vi "CliCommandReceived.vi"(8 "error in (no error)":errorcluster, 10 "CommandReceived":refnum<class "CommandReceived.lvclass">, 11 "Controller in":refnum<class "Controller.lvclass">) -> (0 "error out":errorcluster, 3 "Controller out":refnum<class "Controller.lvclass">)   [LabVIEW 2022 SP3, in "Controller.lvlib" / "Controller.lvclass"]
uses:
  Controller.lvclass
  Cli/CommandReceived/CommandReceived.lvclass
  Cli/CommandReceived/CommandReceived.lvclass/CommandReceived.ctl
  ArgumentParser/Source/ParsedData/ParsedData.lvclass/ParsedData.ctl
  Cli/CommandReceived/Read ParsedData.vi
  ArgumentParser/Source/ParsedData/Read Arguments.vi
  ArgumentParser/Source/ParsedData/ParsedData.lvclass
  Controller.lvclass/Controller.ctl
  ArgumentParser/Source/ParsedData/_Arguments.ctl
  Cli/Cli Messages/WriteToStdOut Msg/WriteToStdOut Msg.lvclass
  Tcp/DataReceived/DataReceived.lvclass
panel:
  out "Arguments":T1
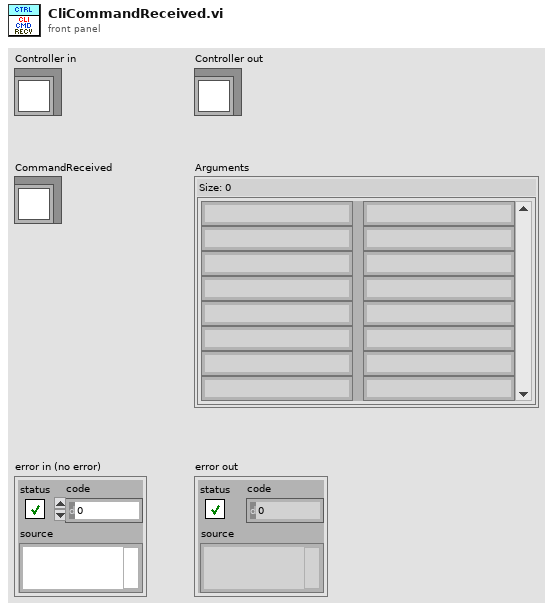
[diagram p1: front panel]
types:
  T1 = typedef "ArgumentParser.lvlib/ParsedData.lvclass/_Arguments.ctl" = map{string, string}
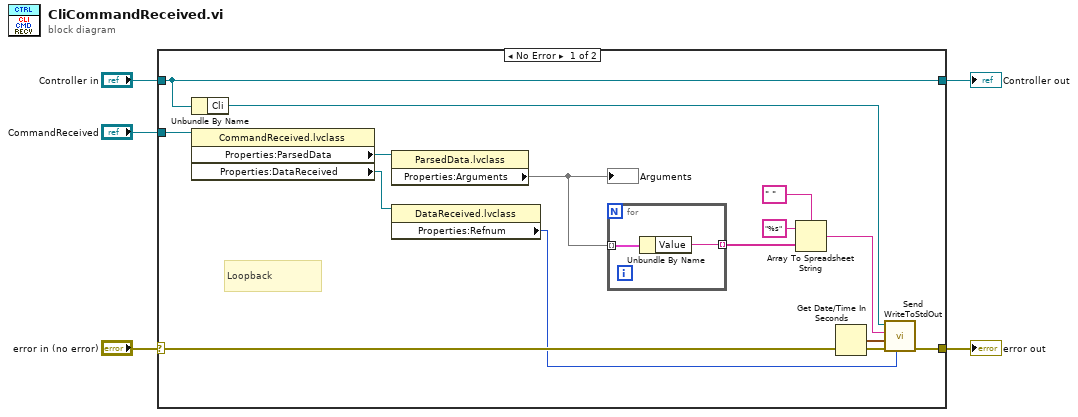
[diagram p0: block diagram]
diagram:
  n1 = case shown="No Error" "error in (no error)" {
    selector: "error in (no error)" -> [w16 w23]
    tunnel: "CommandReceived" -> [w19 _]
    tunnel: [w15 w23] -> w3
    tunnel: "Controller in" -> [w17 w22]
    tunnel: [w17 w22] -> w1
    frame No Error {
      # "Loopback"
      n2 = Unbundle By Name(w17) -> ("Cli"=w14:refnum<class "Message Enqueuer.lvclass">)
      n3 = property class="CommandReceived.lvclass"(reference=w19) -> ("Properties:ParsedData"=w18:refnum<class "ParsedData.lvclass">, "Properties:DataReceived"=w7:refnum<class "DataReceived.lvclass">)  [unwired: 1 in, 2 out]
      n4 = property class="ParsedData.lvclass"(reference=w18) -> ("Properties:Arguments"=w13:T1)  [unwired: 1 in, 2 out]
      "Arguments" <- w13
      n5 = property class="DataReceived.lvclass"(reference=w7) -> ("Properties:Refnum"=w6:u64)  [unwired: 1 in, 2 out]
      n6 = for {
        tunnel: w13 -> [w21] mode=indexing
        tunnel: [w20] -> w12 mode=indexing
        n7 = Unbundle By Name(w21) -> ("Value"=w20:string)
      }
      n8 = Array To Spreadsheet String(delimiter (Tab)=" ", array=w12, 3:"%s" ("format string")) -> (spreadsheet string=w9:string)
      n9 = Get Date/Time In Seconds() -> (seconds since 1Jan1904=w8:timestamp)
      n10 = call "Send WriteToStdOut.vi"("Refnum"=w6, "error in (no error)"=w16, "TimeStamp"=w8, "Data"=w9, "Message Enqueuer"=w14) -> ("error out"=w15:errorcluster)  [unwired: 5 in, 1 out]
    }
    frame Error {
    }
  }
  "error out" <- w3
  "Controller out" <- w1
